vi "Delete_Internal_TargetFileDir_On_Error.vi"(8 "error in (no error)":errorcluster, 10 "override Mac support directory preservation":bool, 11 "Build in":refnum<class "AB_PackedLibrary.lvclass">) -> (0 "error out":errorcluster, 3 "Build out":refnum<class "AB_PackedLibrary.lvclass">)   [LabVIEW 2020, in "AB_PackedLibrary.lvclass"]
uses:
  <vilib>/AppBuilder/AB_Classes/PackedLib/AB_PackedLibrary.lvclass
  <vilib>/AppBuilder/AB_Classes/PackedLib/AB_PackedLibrary.lvclass/AB_PackedLibrary.ctl
  <vilib>/AppBuilder/AB_Classes/TargetFile/AB_Targetfile.lvclass
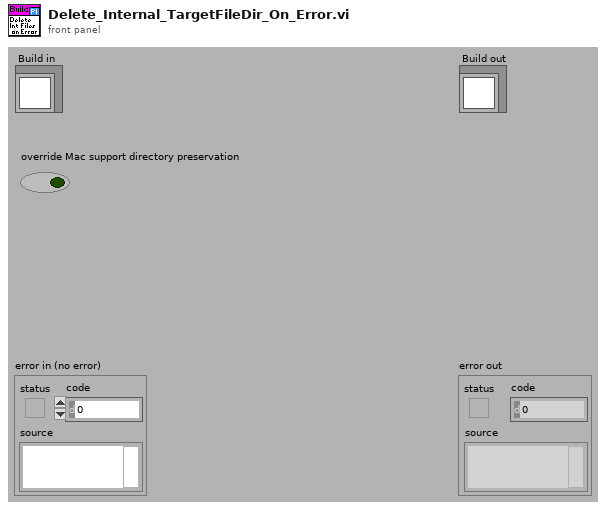
[diagram p1: front panel]
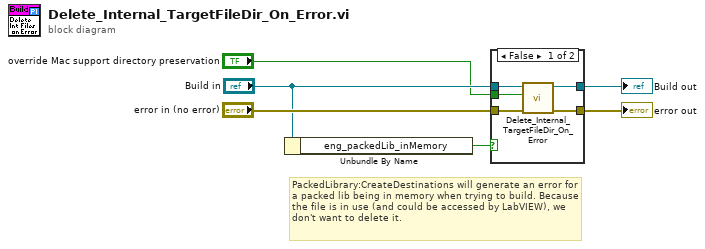
[diagram p0: block diagram]
diagram:
  # "PackedLibrary:CreateDestinations will generate an error for a packed lib being in memory when trying to build. Because the file is in use (and could be accessed by LabVIEW), we don't want to delete it."
  n1 = Unbundle By Name("Build in") -> ("eng_packedLib_inMemory"=w2:bool)
  n2 = case shown="False" w2 {
    tunnel: [w11 w12] -> w6
    tunnel: [w10 w13] -> w5
    tunnel: "error in (no error)" -> [w9 w12]
    tunnel: "Build in" -> [w8 w13]
    tunnel: "override Mac support directory preservation" -> [w7 _]
    frame False {
      n3 = call-parent "Delete_Internal_TargetFileDir_On_Error.vi"("error in (no error)"=w9, "override Mac support directory preservation"=w7, "Build in"=w8) -> ("error out"=w11:errorcluster, "Build out"=w10:refnum<class "AB_PackedLibrary.lvclass">)  [unwired: 7 in]
    }
    frame True {
    }
  }
  "error out" <- w6
  "Build out" <- w5
